vi "TouchPanel.Global.vi"() -> ()   [LabVIEW 2015]
panel:
  out "Current VI ref":refnum<vi>
  in  "TouchPanel active":bool
  in  "Current screen name":string
  in  "Date":string
  in  "Version":string="0.0"
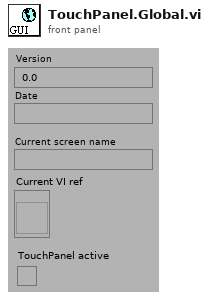
[diagram p1: front panel]
diagram:
